vi "PH_PILS.PC _GUILessTags.vi"(0 "i ref in":refnum<vi>, 2 "serviceName":string, 3 "Value":i32, 5 "error IO":errorcluster) -> (14 "i ref out":refnum<vi>, 19 "error out":errorcluster)   [LabVIEW 2014, in "PH_PILS.lvlib"]
doc: "This VI sets the incoming tag values to own attributes."
uses:
  PH_PILS.lvlib
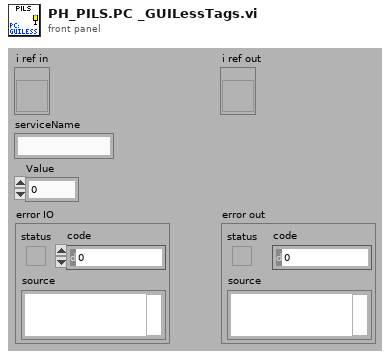
[diagram p1: front panel]
types:
  T1 = typedef "PH_PILS.lvlib/PH_PILS.i attribute.ctl" = cluster{"Boolean":cluster{"GUI Ref":refnum<vi>, "Status":i32}[], "GUI Refs Exp. Shutters":cluster{"1":refnum<vi>, "2":refnum<vi>, "3":refnum<vi>, "4":refnum<vi>}, "Tristate2Run GUI Refs":refnum<vi>[], "EO-Likes":cluster{"GUI Ref":refnum<vi>, "Status":i32}[], "Operation Mode":cluster{"Operation Mode":T2, "GUI":cluster{"Ref State":refnum<vi>, "Ref":refnum<vi>}, "Servicemode":cluster{"Tagname":string, "Status":i32}, "Labormode":cluster{"Tagname":string, "Status":i32}, "Searchmode":cluster{"Tagname":string, "Status":i32}, "Shotmode":cluster{"Tagname":string, "Status":i32}}, "Submode":cluster{"Submode":T3, "GUI":cluster{"Ref State":refnum<vi>, "Ref":refnum<vi>}, "Submode":cluster{"Tagname":string, "Status":i32}}, "Experiment":cluster{"Experiment":enum16{"unknown", "intern", "4 (Z6)", "3", "2", "1"}, "GUI":cluster{"Ref State":refnum<vi>, "Ref":refnum<vi>}, "intern":cluster{"Tagname":string, "Status":i32}, "Exp 4":cluster{"Tagname":string, "Status":i32}, "Exp 3":cluster{"Tagname":string, "Status":i32}, "Exp 2":cluster{"Tagname":string, "Status":i32}, "Exp 1":cluster{"Tagname":string, "Status":i32}}, "TristateNormal":cluster{"GUI Ref":refnum<vi>, "Status":i32}[], "Door Tags":cluster{"GUI Ref":refnum<vi>, "Status":i32}[], "GUIlessTags":cluster{"Name":string, "Status":i32}[], "Beamline GUI Refs":refnum<vi>[], "Special Boolean":cluster{"GUI Ref":refnum<vi>, "Status":i32}[], "Laserpower":cluster{"GUI Ref":refnum<vi>, "Status":i32}[], "Shutter":cluster{"GUI Ref":refnum<vi>, "Status":i32}[], "Tristate EO Like":cluster{"GUI Ref":refnum<vi>, "Status":i32}[], "PP":cluster{"GUI Ref":refnum<vi>, "Status":i32, "Head Ref":refnum<vi>, "Slider Ref":refnum<vi>}[], "Switch Knobs":cluster{"GUI Ref":refnum<vi>, "Status":i32}[], "Latch Knob GUI Refs":refnum<vi>[], "FailureCounter":i32, "Enabled Status":cluster{"Laser":i32, "PreAmp":i32, "MainAmp":i32}, "Mercury":refnum<vi>, "Instance Rods":string, "Logfile":path, "Beckhoff-Instance Internal":string, "Beckhoff-Instance External":string, "Enabling Rights":cluster{"Name":string, "Password":string, "PA?":bool, "MA?":bool, "Exp?":bool}[]}
  T2 = typedef "PH_PILS.lvlib/PH_PILS.Operation Mode.ctl" = enum16{"unknown", "Service", "Labor", "Search", "Shot"}
  T3 = typedef "PH_PILS.lvlib/PH_PILS.Submode.ctl" = enum16{"unknown", "HV-Normal", "HV-Test"}
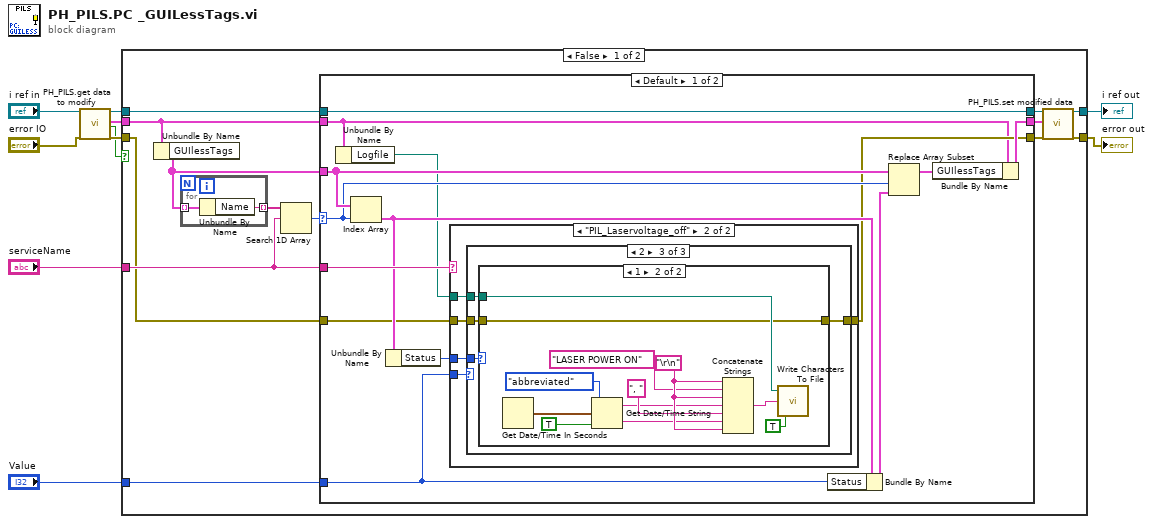
[diagram p0: block diagram]
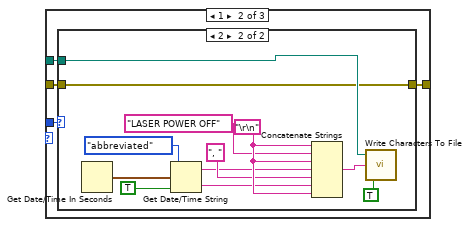
[diagram p4: hidden frame]
diagram:
  n1 = call "PH_PILS.get data to modify.vi"("i ref in"="i ref in", "error in (no error)"="error IO") -> ("i ref out"=w4:refnum<vi>, "i attribute"=w3:T1, "timed out"=w6:bool, "error out"=w7:errorcluster)  [unwired: 14 in]
  n2 = case shown="False" w6 {
    tunnel: w3 -> [w18 _]
    tunnel: w4 -> [w12 w85]
    tunnel: [w23 w85] -> w5
    tunnel: w7 -> [w14 w84]
    tunnel: [w22 w84] -> w8
    tunnel: "Value" -> [w16 _]
    tunnel: "serviceName" -> [w15 _]
    frame False {
      n3 = Unbundle By Name(w18) -> ("GUIlessTags"=w19:cluster{"Name":string, "Status":i32}[])
      n4 = for {
        tunnel: w19 -> [w83] mode=indexing
        tunnel: [w82] -> w21 mode=indexing
        n5 = Unbundle By Name(w83) -> ("Name"=w82:string)
      }
      n6 = Search 1D Array(1D array=w21, element=w15) -> (index of element=w20:i32)  [unwired: 1 in]
      n7 = case shown="Default" w20 {
        selector: w20 -> [w32 _]
        tunnel: w19 -> [w35 _]
        tunnel: w18 -> [w27 w81]
        tunnel: [w36 w81] -> w17
        tunnel: w16 -> [w31 _]
        tunnel: w15 -> [w33 _]
        tunnel: w14 -> [w25 w80]
        tunnel: [w28 w80] -> w13
        tunnel: w12 -> [w24 w79]
        tunnel: [w24 w79] -> w11
        frame Default {
          n8 = Unbundle By Name(w27) -> ("Logfile"=w26:path)
          n9 = Index Array(array=w35, index=w32) -> (element=w30:cluster{"Name":string, "Status":i32})
          n10 = Unbundle By Name(w30) -> ("Status"=w29:i32)
          n11 = case shown="\"PIL_Laservoltage_off\"" w33 {
            tunnel: w31 -> [_ w43]
            tunnel: w29 -> [_ w42]
            tunnel: w26 -> [_ w41]
            tunnel: w25 -> [w38 w40]
            tunnel: [w38 w39] -> w28
            frame Default {
            }
            frame "PIL_Laservoltage_off" {
              n12 = case shown="2" w43 {
                tunnel: w42 -> [_ w48 w65]
                tunnel: w41 -> [_ w47 w64]
                tunnel: w40 -> [w44 w46 w63]
                tunnel: [w44 w45 w62] -> w39
                frame Default {
                }
                frame 1 {
                  n13 = case shown="2" w48 {
                    tunnel: w47 -> [_ w52]
                    tunnel: w46 -> [w49 w50]
                    tunnel: [w49 w50] -> w45
                    frame Default {
                    }
                    frame 2 {
                      w61 = "\r\n"
                      n14 = Get Date/Time In Seconds() -> (seconds since 1Jan1904=w55:timestamp)
                      n15 = Get Date/Time String(date format (0)=enum16{"short", "long", "abbreviated"}."abbreviated", seconds (now)=w55, want seconds? (F)=TRUE) -> (date string=w57:string, time string=w58:string)
                      n16 = Concatenate Strings(w61, "LASER POWER OFF" ("string"), w61, w57, ", ", w58, w61) -> (w53:string)
                      n17 = call <vilib>:"Write Characters To File.vi"("append to file? (new file:F)"=TRUE, "character string"=w53, "file path (dialog if empty)"=w52) -> ()  [unwired: 2 in, 1 out]
                    }
                  }
                }
                frame 2 {
                  n18 = case shown="1" w65 {
                    tunnel: w64 -> [_ w69]
                    tunnel: w63 -> [w66 w68]
                    tunnel: [w66 w68] -> w62
                    frame Default {
                    }
                    frame 1 {
                      w78 = "\r\n"
                      n19 = Get Date/Time In Seconds() -> (seconds since 1Jan1904=w72:timestamp)
                      n20 = Get Date/Time String(date format (0)=enum16{"short", "long", "abbreviated"}."abbreviated", seconds (now)=w72, want seconds? (F)=TRUE) -> (date string=w74:string, time string=w75:string)
                      n21 = Concatenate Strings(w78, "LASER POWER ON" ("string"), w78, w74, ", ", w75, w78) -> (w70:string)
                      n22 = call <vilib>:"Write Characters To File.vi"("append to file? (new file:F)"=TRUE, "character string"=w70, "file path (dialog if empty)"=w69) -> ()  [unwired: 2 in, 1 out]
                    }
                  }
                }
              }
            }
          }
          n23 = Bundle By Name(cluster=w30, "Status"=w31) -> (w34:cluster{"Name":string, "Status":i32})
          n24 = Replace Array Subset(array=w35, new element=w34, index=w32) -> (w37:cluster{"Name":string, "Status":i32}[])
          n25 = Bundle By Name(cluster=w27, "GUIlessTags"=w37) -> (w36:T1)
        }
        frame -1 {
        }
      }
      n26 = call "PH_PILS.set modified data.vi"("i ref in"=w11, "i attribute"=w17, "error in (no error)"=w13) -> ("i ref out"=w23:refnum<vi>, "error out"=w22:errorcluster)  [unwired: 15 in]
    }
    frame True {
    }
  }
  "error out" <- w8
  "i ref out" <- w5
